vi "Launch.vi"(8 "error in (no error)":errorcluster, 11 "TCP_Server in":refnum<class "TCP_Server.lvclass">) -> (0 "error out":errorcluster, 3 "TCP_Server out":refnum<class "TCP_Server.lvclass">)   [LabVIEW 2013, in "TCP_Server.lvclass"]
uses:
  TCP_Server.lvclass
  TCP_Server.lvclass/TCP_Server.ctl
panel:
  in  "port":u16=6340
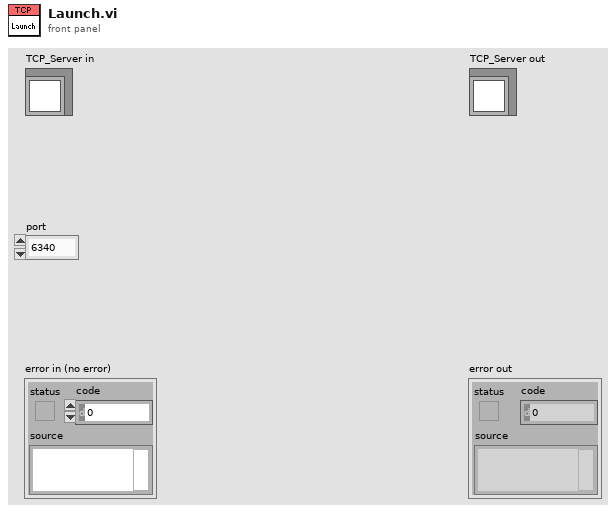
[diagram p1: front panel]
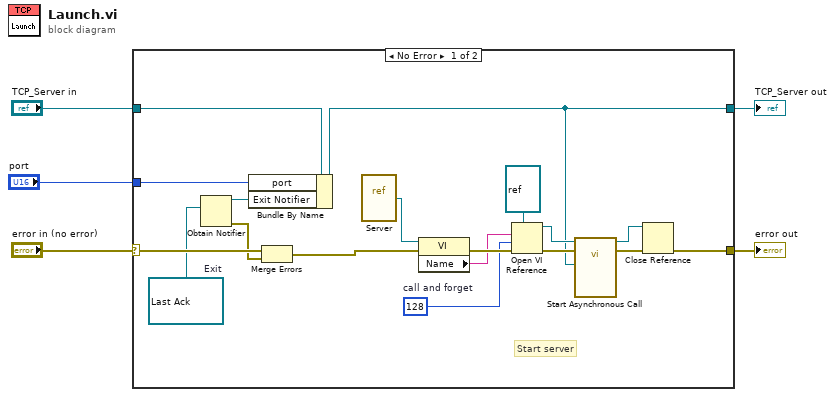
[diagram p0: block diagram]
diagram:
  n1 = case shown="No Error" "error in (no error)" {
    selector: "error in (no error)" -> [w10 w25]
    tunnel: [w11 w25] -> w4
    tunnel: [w12 w24] -> w2
    tunnel: "TCP_Server in" -> [w23 w24]
    tunnel: "port" -> [w22 _]
    frame No Error {
      w9 = refnum<notifier> refnum  # Exit
      w13 = 128  # call and forget
      # "Start server"
      n2 = Obtain Notifier(notification data type=w9) -> (notifier out=w8:refnum<notifier>, error out=w6:errorcluster)  [unwired: 3 in, 1 out]
      n3 = Bundle By Name(cluster=w23, "port"=w22, "Exit Notifier"=w8) -> (w12:refnum<class "TCP_Server.lvclass">)
      n4 = Merge Errors(w10, w6) -> (w7:errorcluster)
      n5 = vi-ref "Server.vi"() -> (w19:refnum<vi>)
      n6 = property class="VI"(reference=w19, error in=w7) -> (error out=w21:errorcluster, "Name"=w20:string)  [unwired: 1 out]
      n7 = Open VI Reference(type specifier VI Refnum (for type only)=refnum<vi> refnum, vi path=w20, options=w13, error in (no error)=w21) -> (vi reference=w15:refnum<vi>, error out=w16:errorcluster)  [unwired: 2 in]
      n8 = call-by-ref "Start Asynchronous Call"(reference=w15, error in=w16, "TCP_Server in"=w12) -> (reference out=w18:refnum<vi>, error out=w17:errorcluster)  [unwired: 9 in, 2 out]
      n9 = Close Reference(reference=w18, error in (no error)=w17) -> (error out=w11:errorcluster)
    }
    frame Error {
    }
  }
  "error out" <- w4
  "TCP_Server out" <- w2
